vi "Detect Rectangle - Main Video Processing.vi"() -> ()   [LabVIEW 2014]
uses:
  <vilib>/vision/Pattern Matching.llb/IMAQ Curve Parameters.ctl
  <vilib>/vision/Shape Detection.llb/ShapeDetectionMatchOptions.ctl
  <vilib>/vision/Pattern Matching.llb/IMAQ Match Range Setting.ctl
  Others (.ctl)/Control cluster.ctl
  Global.vi
  <vilib>/vision/NI_Vision_Development_Module.lvlib
panel:
  in  "Curve Parameters":T1={"Extraction Mode"=0, "Edge Threshold"=75, "Edge Filter Size"=1, "Min Length"=25, "Row Search Step Size"=15, "Col Search Step Size"=15, "Max Endpoint Gap"=10, "Closed"=FALSE, "Subpixel"=FALSE} {"Extraction Mode" items=["Normal", "Uniform Regions"]; "Edge Filter Size" items=["Fine", "Normal", "Contour Tracing"]; "Max Endpoint Gap" min=0; "Col Search Step Size" min=1 max=255 step=1; "Row Search Step Size" min=1 max=255 step=1; "Min Length" min=0; "Edge Threshold" min=1 max=350 step=1}
  out "Image":T2(plugin-control)
  out "error out 2":errorcluster
  out "error out":errorcluster
  out "Rectangles":T3(array[cluster]) {"Corners"."Y" format="%.2f"; "Corners"."X" format="%.2f"}
  in  "Minimum match score":dbl
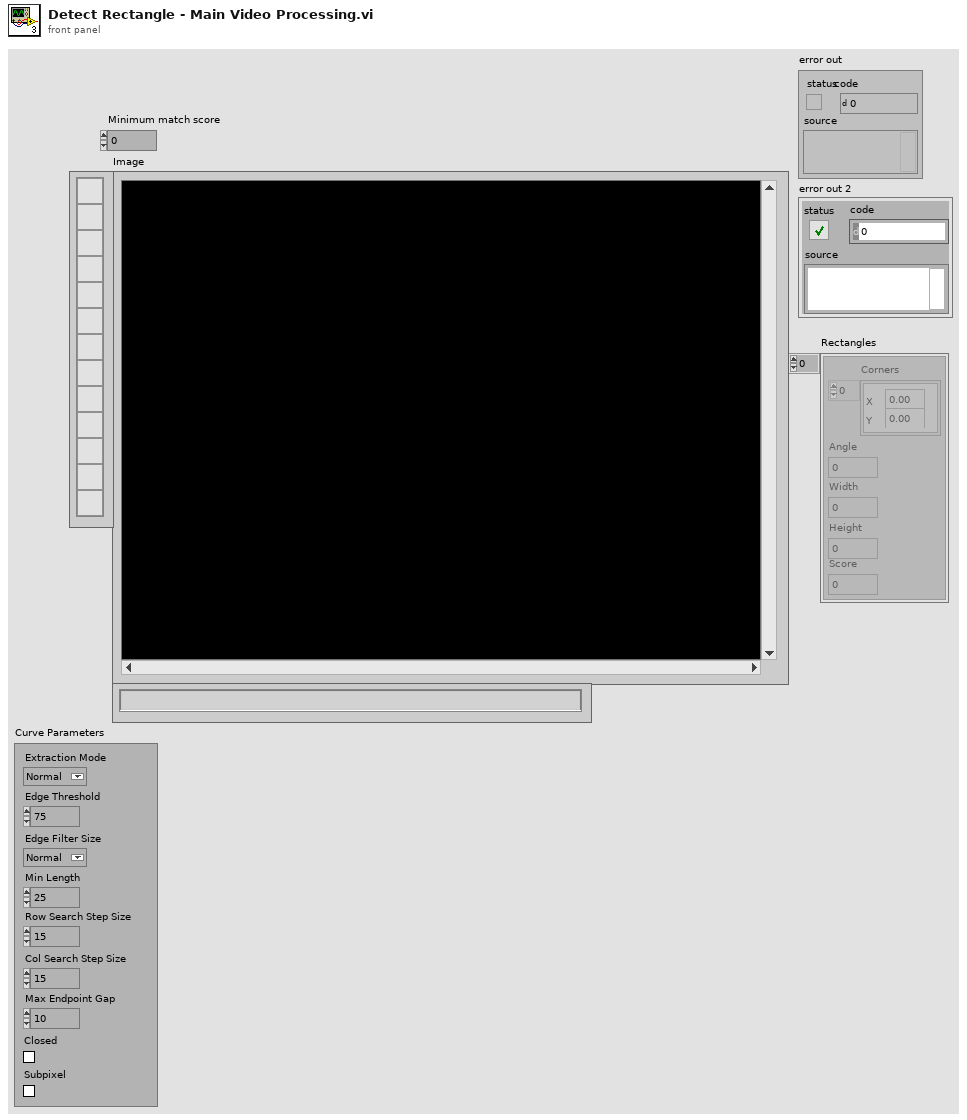
[diagram p1: front panel]
types:
  T1 = typedef "IMAQ Curve Parameters.ctl" = cluster{"Extraction Mode":u32, "Edge Threshold":i32, "Edge Filter Size":u32, "Min Length":i32, "Row Search Step Size":i32, "Col Search Step Size":i32, "Max Endpoint Gap":i32, "Closed":bool, "Subpixel":bool}
  T2 = typedef "IMAQ Image.ctl" = refnum<image>
  T3 = cluster{"Corners":cluster{"X":sgl, "Y":sgl}[], "Angle":dbl, "Width":dbl, "Height":dbl, "Score":dbl}[]
  T4 = typedef "Control cluster.ctl" = cluster{"Roll":sgl, "Pitch":sgl, "Vertical Speed":sgl, "Yaw Speed":sgl}
  T5 = typedef "ShapeDetectionMatchOptions.ctl" = cluster{"Rotation":bool, "Scale":bool, "Occlusion":bool, "Range Settings":T6[]}
  T6 = typedef "IMAQ Match Range Setting.ctl" = cluster{"Match Constraints":u32, "Min":dbl, "Max":dbl}
  T7 = cluster{"Min Width":dbl, "Max Width":dbl, "Min Height":dbl, "Max Height":dbl}
  T8 = typedef "Image Type" = u32
  T9 = cluster{"Corners":cluster{"X":sgl, "Y":sgl}[], "Angle":dbl, "Width":dbl, "Height":dbl, "Score":dbl}
  T10 = cluster{"Corners[0]":cluster{"X":sgl, "Y":sgl}, "Corners[1]":cluster{"X":sgl, "Y":sgl}, "Corners[2]":cluster{"X":sgl, "Y":sgl}, "Corners[3]":cluster{"X":sgl, "Y":sgl}, "Corners[4]":cluster{"X":sgl, "Y":sgl}, "Corners[5]":cluster{"X":sgl, "Y":sgl}, "Corners[6]":cluster{"X":sgl, "Y":sgl}, "Corners[7]":cluster{"X":sgl, "Y":sgl}, "Corners[8]":cluster{"X":sgl, "Y":sgl}}
  T11 = cluster{"Corners[0]":cluster{"X":sgl, "Y":sgl}, "Corners[1]":cluster{"X":sgl, "Y":sgl}, "Corners[2]":cluster{"X":sgl, "Y":sgl}, "Corners[3]":cluster{"X":sgl, "Y":sgl}}
  T12 = cluster{"[0]":cluster{"X":sgl, "Y":sgl}, "[1]":cluster{"X":sgl, "Y":sgl}, "[2]":cluster{"X":sgl, "Y":sgl}, "[3]":cluster{"X":sgl, "Y":sgl}, "[4]":cluster{"X":sgl, "Y":sgl}, "[5]":cluster{"X":sgl, "Y":sgl}, "[6]":cluster{"X":sgl, "Y":sgl}, "[7]":cluster{"X":sgl, "Y":sgl}, "[8]":cluster{"X":sgl, "Y":sgl}}
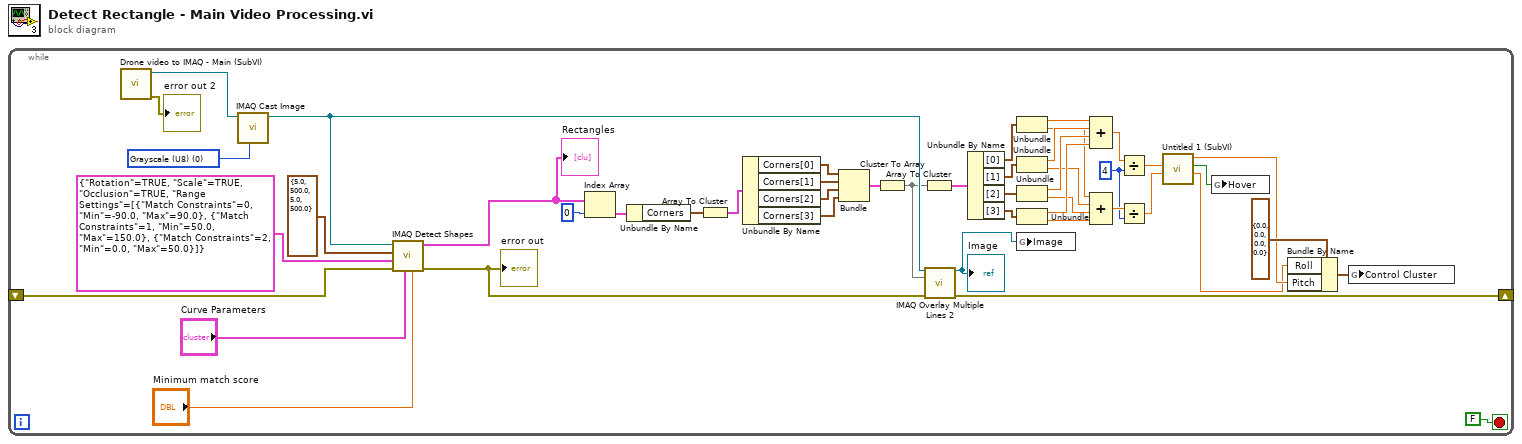
[diagram p0: block diagram]
diagram:
  n1 = while {
    shift-right: [w34] -> _
    shift-left: _ -> [w43]
    stop <- FALSE stop-if-true
    w8 = 4
    w40 = T8 0 items=["Grayscale (U8)", "Grayscale (I16)", "Grayscale (SGL)", "Complex (CSG)", "RGB (U32)", "HSL (U32)", "RGB (U64)", "Grayscale (U16)"] ("Image Type")
    n2 = call "Drone video to IMAQ - Main (SubVI).vi"() -> ("error out"=→"error out 2":errorcluster, "raw image"=w41:T2)  [unwired: 10 in]
    n3 = call "IMAQ Cast Image"("Image Type"=w40, "Image Src"=w41) -> ("Image Dst Out"=w37:T2)  [unwired: 8 in, 1 out]
    n4 = call-poly "IMAQ Detect Shapes"("Minimum match score"="Minimum match score", "Curve Parameters"="Curve Parameters", "error in (no error)"=w43, "Match Options"=T5 {"Rotation"=TRUE, "Scale"=TRUE, "Occlusion"=TRUE, "Range Settings"=[{"Match Constraints"=0, "Min"=-90.0, "Max"=90.0}, {"Match Constraints"=1, "Min"=50.0, "Max"=150.0}, {"Match Constraints"=2, "Min"=0.0, "Max"=50.0}]}, "Rectangle Descriptor"=T7 {"Min Width"=5.0, "Max Width"=500.0, "Min Height"=5.0, "Max Height"=500.0}, "Image"=w37) -> ("error out"=w35:errorcluster, "Rectangles"=w39:T3)  [unwired: 3 in, 1 out]
    "Rectangles" <- w39
    "error out" <- w35
    n5 = Index Array(array=w39, index=0) -> (element=w36:T9)
    n6 = Unbundle By Name(w36) -> ("Corners"=w33:cluster{"X":sgl, "Y":sgl}[])
    n7 = Array To Cluster(array=w33) -> (cluster=w32:T10)
    n8 = Unbundle By Name(w32) -> ("Corners[0]"=w29:cluster{"X":sgl, "Y":sgl}, "Corners[1]"=w30:cluster{"X":sgl, "Y":sgl}, "Corners[2]"=w31:cluster{"X":sgl, "Y":sgl}, "Corners[3]"=w28:cluster{"X":sgl, "Y":sgl})
    n9 = Bundle("Corners[0]"=w29, "Corners[1]"=w30, "Corners[2]"=w31, "Corners[3]"=w28) -> (w27:T11)  [unwired: 1 in]
    n10 = Cluster To Array(cluster=w27) -> (array=w24:cluster{"X":sgl, "Y":sgl}[])
    n11 = Array To Cluster(array=w24) -> (cluster=w23:T12)
    n12 = call "IMAQ Overlay Multiple Lines 2"("Image"=w37, "Line End Points"=w24, "error in (no error)"=w35) -> ("Image Out"=w25:T2, "error out"=w34:errorcluster)  [unwired: 11 in]
    "Image" <- w25
    n13 = Unbundle By Name(w23) -> ("[0]"=w19:cluster{"X":sgl, "Y":sgl}, "[1]"=w20:cluster{"X":sgl, "Y":sgl}, "[2]"=w21:cluster{"X":sgl, "Y":sgl}, "[3]"=w22:cluster{"X":sgl, "Y":sgl})
    n14 = Unbundle(w19) -> ("X"=w18:sgl, "Y"=w11:sgl)
    n15 = Unbundle(w20) -> ("X"=w17:sgl, "Y"=w12:sgl)
    n16 = Unbundle(w21) -> ("X"=w16:sgl, "Y"=w13:sgl)
    n17 = Unbundle(w22) -> ("X"=w15:sgl, "Y"=w14:sgl)
    n18 = global write "Global.vi" "Image"(w25) -> ()
    n19 = Compound Arithmetic op=ADD(w18, w17, w16, w15) -> (w10:sgl)
    n20 = Compound Arithmetic op=ADD(w11, w12, w13, w14) -> (w9:sgl)
    n21 = Divide(x=w10, y=w8) -> (x/y=w7:sgl)
    n22 = Divide(x=w9, y=w8) -> (x/y=w6:sgl)
    n23 = call "Untitled 1 (SubVI).vi"("X"=w6, "Y"=w7) -> ("Roll"=w2:dbl, "Hover"=w1:bool, "Pitch"=w3:dbl)  [unwired: 7 in]
    n24 = global write "Global.vi" "Hover"(w1) -> ()
    n25 = Bundle By Name(cluster=T4 {"Roll"=0.0, "Pitch"=0.0, "Vertical Speed"=0.0, "Yaw Speed"=0.0} ("Control Cluster"), "Roll"=w2, "Pitch"=w3) -> (w4:T4)
    n26 = global write "Global.vi" "Control Cluster"(w4) -> ()
  }
